vi "Write VI Store.vi"(8 "error in (no error)":errorcluster, 10 "VI App Store.lvlib:VIStore.lvclass":refnum<class "VIStore.lvclass">, 11 "Settings in":refnum<class "Settings.lvclass">) -> (0 "error out":errorcluster, 3 "Settings out":refnum<class "Settings.lvclass">)   [LabVIEW 2015, in "Item Actor.lvlib" / "Settings.lvclass"]
uses:
  Settings.lvclass
  VI Store/VIStore Actor/VIStore.lvclass
  Settings.lvclass/Settings.ctl
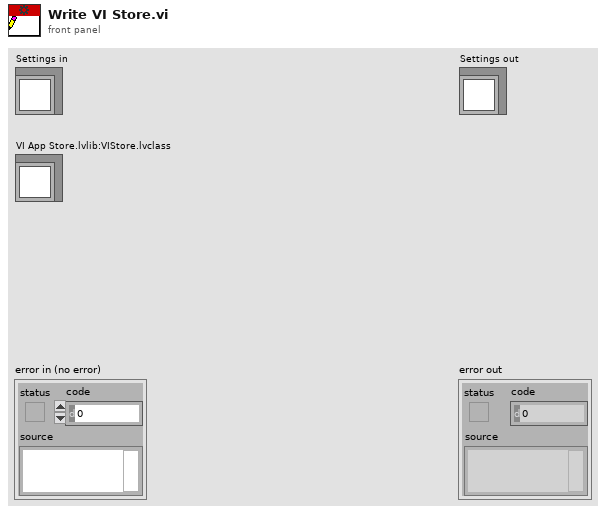
[diagram p1: front panel]
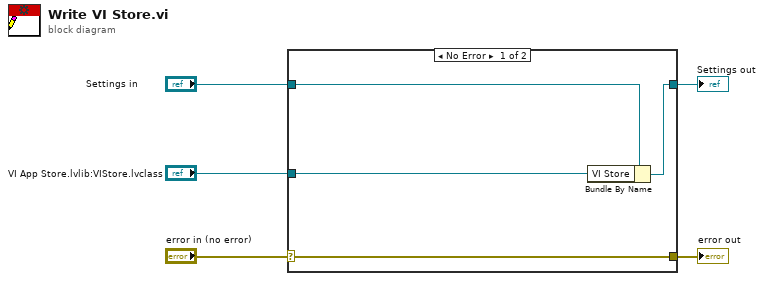
[diagram p0: block diagram]
diagram:
  n1 = case shown="No Error" "error in (no error)" {
    selector: "error in (no error)" -> [w9 w10]
    tunnel: [w9 w10] -> w4
    tunnel: [w7 w11] -> w2
    tunnel: "Settings in" -> [w8 w11]
    tunnel: "VI App Store.lvlib:VIStore.lvclass" -> [w6 _]
    frame No Error {
      n2 = Bundle By Name(cluster=w8, "VI Store"=w6) -> (w7:refnum<class "Settings.lvclass">)
    }
    frame Error {
    }
  }
  "error out" <- w4
  "Settings out" <- w2
